vi "scan string.vi"() -> ()   [LabVIEW 2017]
panel:
  in  "input string":string
  out "remaining string":string
  out "output 1":dbl
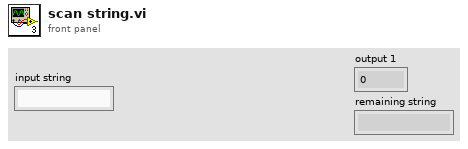
[diagram p1: front panel]
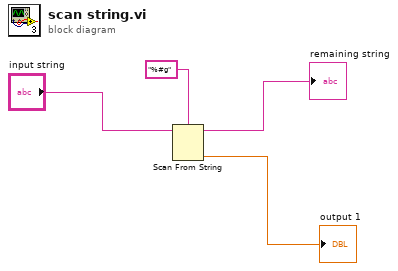
[diagram p0: block diagram]
diagram:
  n1 = Scan From String(format string="%#g", input string="input string") -> (remaining string=→"remaining string":string, output 1=→"output 1":dbl)  [unwired: 3 in, 2 out]
